vi "Move Sort Label.vi"(8 "error in (no error)":errorcluster, 10 "Target Label":refnum<vi>, 11 "Endpoint Configuration Page Controls":T1) -> (0 "error out":errorcluster)   [LabVIEW 2017, in "SLSC Switch System Explorer.lvlib"]
uses:
  SLSC Switch System Explorer.lvlib
  Endpoint Configuration Page Controls.ctl
  Shared/UI Common/Sort Button.ctl
  Shared/UI Common/UI Common.lvlib
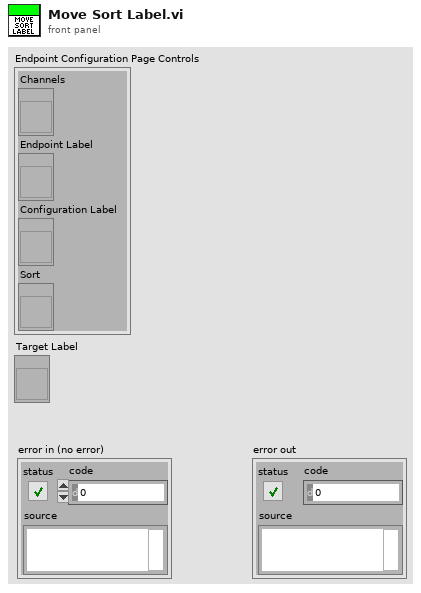
[diagram p1: front panel]
types:
  T1 = typedef "SLSC Switch System Explorer.lvlib/Endpoint Configuration Page Controls.ctl" = cluster{"Channels":refnum<vi>, "Endpoint Label":refnum<vi>, "Configuration Label":refnum<vi>, "Sort":refnum<vi>}
  T2 = typedef "LVPositionTypeDef.ctl" = cluster{"Left":i32, "Top":i32}
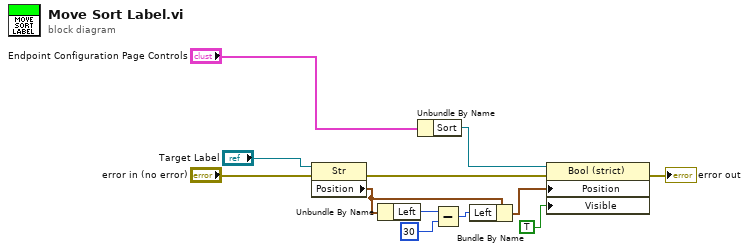
[diagram p0: block diagram]
diagram:
  n1 = property class="Str"(reference="Target Label", error in="error in (no error)") -> (error out=w10:errorcluster, "Position"=w6:T2)  [unwired: 1 out]
  n2 = Unbundle By Name(w6) -> ("Left"=w3:i32)
  n3 = Unbundle By Name("Endpoint Configuration Page Controls") -> ("Sort"=w8:refnum<vi>)
  n4 = Subtract(x=w3, y=30) -> (x-y=w5:i32)
  n5 = Bundle By Name(cluster=w6, "Left"=w5) -> (w9:T2)
  n6 = property class="Bool (strict)"(reference=w8, error in=w10, "Position"=w9, "Visible"=TRUE) -> (error out=→"error out":errorcluster)  [unwired: 1 out]
